vi "TCP Read.vi"(8 "error in":errorcluster, 9 "timeout":i32, 10 "bytes to read":i32, 11 "connection ID":refnum<k5>) -> (0 "error out":errorcluster, 1 "timed out?":bool, 2 "data":u8[](array[numeric]))   [LabVIEW 2013, in "Modbus Library - Advance.lvlib" / "TCP Shared Components.lvlib"]
doc: "This function reads a TCP packet from the bus and checks for errors. It is a wrapper for standard functionality."
uses:
  TCP Shared Components.lvlib
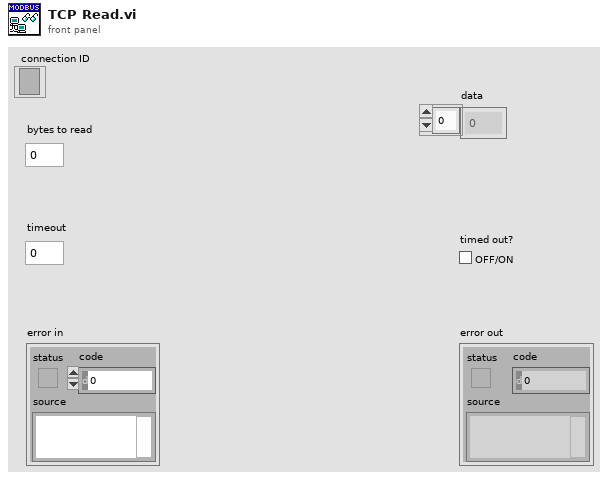
[diagram p1: front panel]
types:
  T1 = enum16{"Standard", "Buffered", "CRLF", "Immediate"}
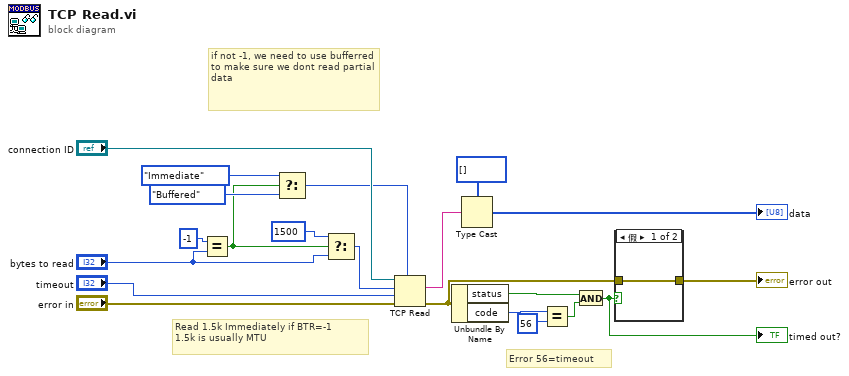
[diagram p0: block diagram]
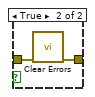
[diagram p2: hidden frame]
diagram:
  # "Read 1.5k Immediately if BTR=-1\n1.5k is usually MTU"
  # "if not -1, we need to use bufferred to make sure we dont read partial data"
  # "Error 56=timeout"
  n1 = Equal?(x=-1, y="bytes to read") -> (x = y?=w4:bool)
  n2 = Select(t=T1."Immediate" ("mode (standard)"), s=w4, f=T1."Buffered" ("mode (standard)")) -> (s? t:f=w6:T1)
  n3 = Select(t=1500, s=w4, f="bytes to read") -> (s? t:f=w2:i32)
  n4 = TCP Read(connection ID="connection ID", bytes to read=w2, error in (no error)="error in", 7:w6, 9:"timeout") -> (data out=w10:string, error out=w5:errorcluster)  [unwired: 1 out]
  n5 = Unbundle By Name(w5) -> ("status"=w13:bool, "code"=w15:i32)
  n6 = Type Cast(type=u8[] [] ("data"), x=w10) -> (*(type *) &x=→"data":u8[])
  n7 = Equal?(x=w15, y=56) -> (x = y?=w12:bool)
  n8 = And(x=w13, y=w12) -> (x .and. y?=w19:bool)
  "timed out?" <- w19
  n9 = case shown="假" w19 {
    tunnel: w5 -> [w22 w24]
    tunnel: [w22 w23] -> w20
    frame False {
    }
    frame True {
      n10 = call <vilib>:"Clear Errors.vi"("error in (no error)"=w24) -> ("error out"=w23:errorcluster)  [unwired: 6 in]
    }
  }
  "error out" <- w20
